vi "Pythagoras.vi"(8 "Motor 2 Coordinate (bottom right)":dbl, 9 "Motor 1 Coordinate (bottom right)":dbl, 10 "Motor 2 Coordinate (top left)":dbl, 11 "Motor 1 Coordinate (top left)":dbl) -> (3 "In Plain Distance":dbl)   [LabVIEW 2018]
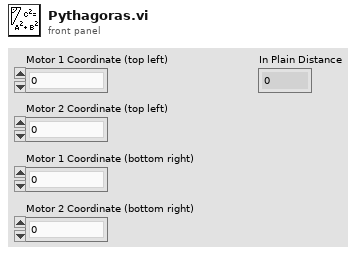
[diagram p1: front panel]
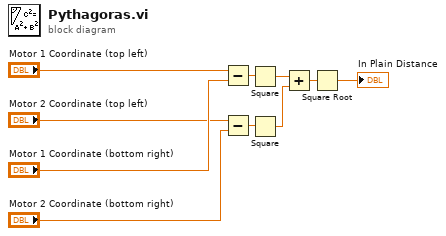
[diagram p0: block diagram]
diagram:
  n1 = Subtract(x="Motor 1 Coordinate (top left)", y="Motor 1 Coordinate (bottom right)") -> (x-y=w6:dbl)
  n2 = Subtract(x="Motor 2 Coordinate (top left)", y="Motor 2 Coordinate (bottom right)") -> (x-y=w5:dbl)
  n3 = Square(x=w6) -> (x^2=w4:dbl)
  n4 = Square(x=w5) -> (x^2=w3:dbl)
  n5 = Add(x=w4, y=w3) -> (x+y=w2:dbl)
  n6 = Square Root(x=w2) -> (sqrt(x)=→"In Plain Distance":dbl)
